vi "FPGA car.vi"() -> ()   [LabVIEW 2019]
doc: "The myRIO v1.1 FPGA Shipping Personality. This personality contains support for:\n- 2 Analog Input Interrupt channel\n- 4 Digital Input Interrupt channel\n- 1 Timer\n- 1 Accelerometer\n- 1 Button\n- 4 LED\n- 10 Analog Input channels with 1 Sample\n- 6 Analog Output channels with 1 Sample\n- 40 Digital I/O channels with 1 Sample\n- 2 I2C channels\n- 4 Encoder channels\n- 6 PWM channels\n- 2 SPI channels"
uses:
  Sub VIs/Utilities/Start Boolean.ctl
  <vilib>/Platform/TimedLoop/XDataNode/timing_clust.ctl
  <vilib>/Platform/TimedLoop/XDataNode/nitl_modes.ctl
  <vilib>/Platform/TimedLoop/XDataNode/wakeup.ctl
  <vilib>/rvi/Emulation/niFpgaGetClockAttributes.vi
  <vilib>/rvi/Emulation/niFpgaSctlEmulationGetInTimedLoop.vi
  <vilib>/rvi/Emulation/niFpgaEmulationReportErrorSimple.vi
  <vilib>/rvi/eio/common/nirviEmuTemplateMethod_errors.vi
  <vilib>/rvi/Emulation/niFpgaProcessEmulError.vi
  <vilib>/rvi/Emulation/niFpgaCriticalErrorInLSC.vi
  <vilib>/eio/EIONode/EIONode.xnode
  <vilib>/Platform/TimedLoop/XDataNode/XDataNode.xnode
  <vilib>/Platform/TimedLoop/XDataNode/XDNodeRunTimeDep.lvlib
panel:
  out "Position 4":i32
  in  "Direction 2":bool
  in  "puls duration us (0-2^16) 2":u32
  in  "Reset 4":bool
  out "Position 3":i32
  in  "Direction":bool
  in  "puls duration us (0-2^16)":u32
  in  "Reset 3":bool
  out "Position 2":i32
  out "Position":i32
  out "arrived 2":bool
  in  "Max_speed half period (us) 2":u16
  in  "Acceleration 2":u16
  in  "Min_speed half period (us) 2":u16
  in  "Soll_pos (Halbschritte) 2":i32
  in  "Reset 2":bool
  out "arrived":bool
  in  "Acceleration":u16
  in  "Max_speed half period (us)":u16
  in  "Min_speed half period (us)":u16
  in  "Reset":bool
  in  "Soll_pos (Halbschritte)":i32
  in  "Duty_counts (0-40)":u16 caption="Count(uSec)"
  out "Time1":u16
  out "Time2":u16
  out "Time 3":u16
  in  "Timeout US":u16
  in  "DO.LED3:0":u8 format="%04b"
  in  "DIO.A_15:8.DIR":u8 format="%08b"
  in  "DIO.A_15:8.OUT":u8 format="%08b"
  in  "SYS.SELECTA":u8 format="%08b"
  out "DIO.A_15:8.IN":u8 format="%08b"
  in  "PWM 2 value (0-1000)":u16
  in  "PWM 1 value (0-1000)":u16
  in  "PWM 0 value (0-1000)":u16
  out "PulseWidth 3":u16
  out "PulseWidth 2":u16
  out "PulseWidth 1":u16
  out "I2C.A.STAT":u8 format="%08b"
  in  "I2C.A.CNTL":u8 format="%08b"
  in  "I2C.A.CNTR":u8=213
  in  "I2C.A.ADDR":u8 format="%08b"
  out "I2C.A.DATI":u8
  in  "I2C.A.DATO":u8
  in  "I2C.A.CNFG":u8=1 format="%08b"
  in  "I2C.A.GO":T1
  out "SYS.AI.RDY":bool
  out "SYS.RDY":bool
  out "ACC.X.VAL":u16
  out "ACC.Y.VAL":u16
  out "SYS.ACC.RDY":bool
  out "ACC.Z.VAL":u16
  # "System"
  # "Onboard Devices"
  # "Connector A"
  # "Accelerometer"
  # "Analog Input"
  # "PWM Output"
  # "PW_Measurement"
  # "I2C Master"
  # "US Measurements"
  # "Stepper Speed"
  # "Stepper Position Freq/Dir"
  # "Led"
  # "Lidar"
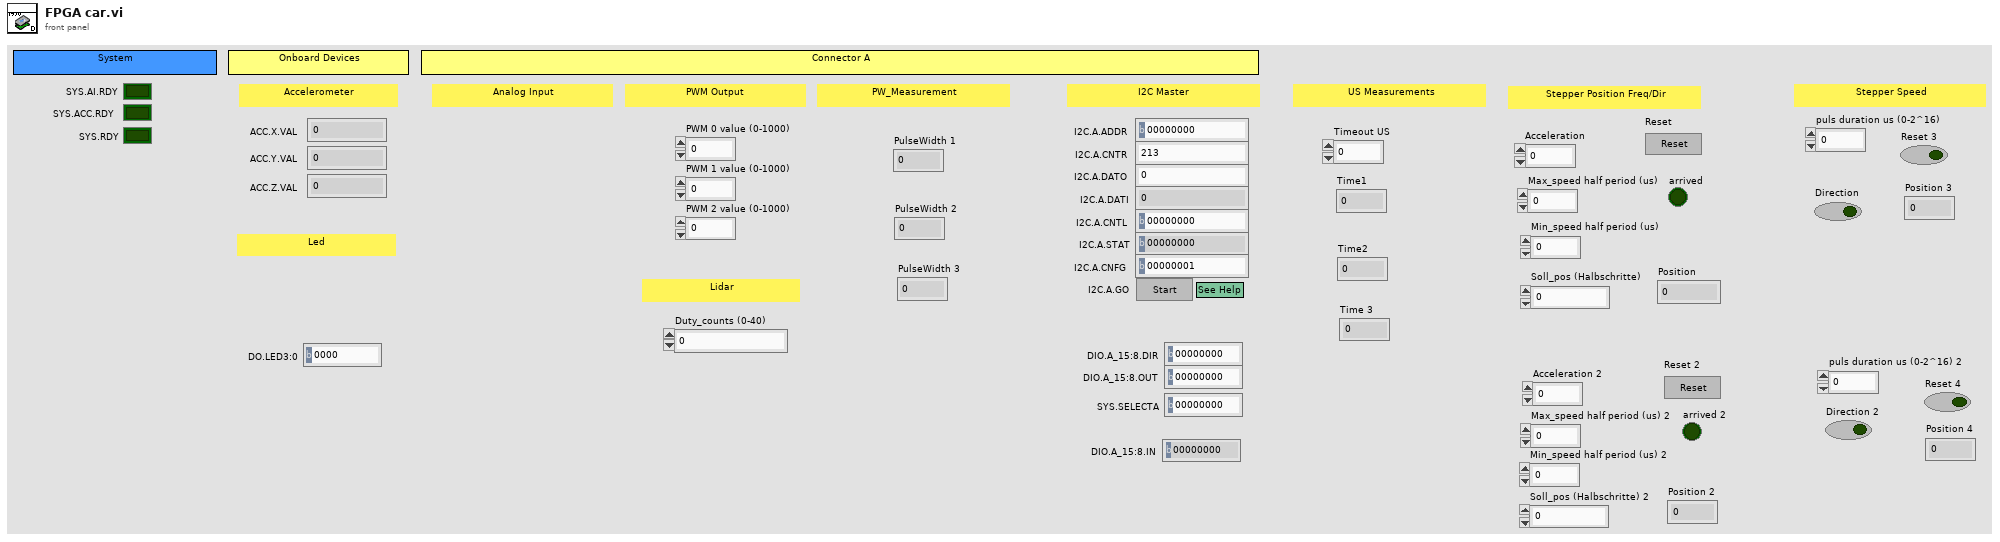
[diagram p1: front panel]
types:
  T1 = typedef "Start Boolean.ctl" = bool
  T2 = typedef "XDNodeRunTimeDep.lvlib/timing_clust.ctl" = cluster{"Expected End [f-1]":u64, "Actual End [f-1]":u64, "Finished Late? [f-1]":bool, "Expected End [i-1]":u64, "Actual End [i-1]":u64, "Finished Late? [i-1]":bool, "Expected Start [i]":u64, "Actual Start [i]":u64, "Expected Start [f]":u64, "Actual Start [f]":u64, "Source Name":string, "Structure Name":string, "Period":i64, "Deadline":i64, "Offset":i64, "Start":i64, "Priority":i32, "Timeout":i32, "Mode":T3, "Wakeup Reason":T4, "Error":errorcluster, "Source Type":string, "Secondary Source Type":string, "Global End Time":u64, "Global Start Time":u64, "Frame Duration":u64, "Iteration Duration":u64, "Assigned CPU":i32, "I/O Scan Engine Mode":u32}
  T3 = typedef "XDNodeRunTimeDep.lvlib/nitl_modes.ctl" = enum32{"No Change", "Process missed periods, maintain original phase", "Discard missed periods, maintain original phase", "Process missed periods, ignore original phase", "Discard missed periods, ignore original phase"}
  T4 = typedef "XDNodeRunTimeDep.lvlib/wakeup.ctl" = enum32{"Normal", "Aborted", "Asynchronous wakeup", "Timing source error", "Timed loop error", "Timeout"}
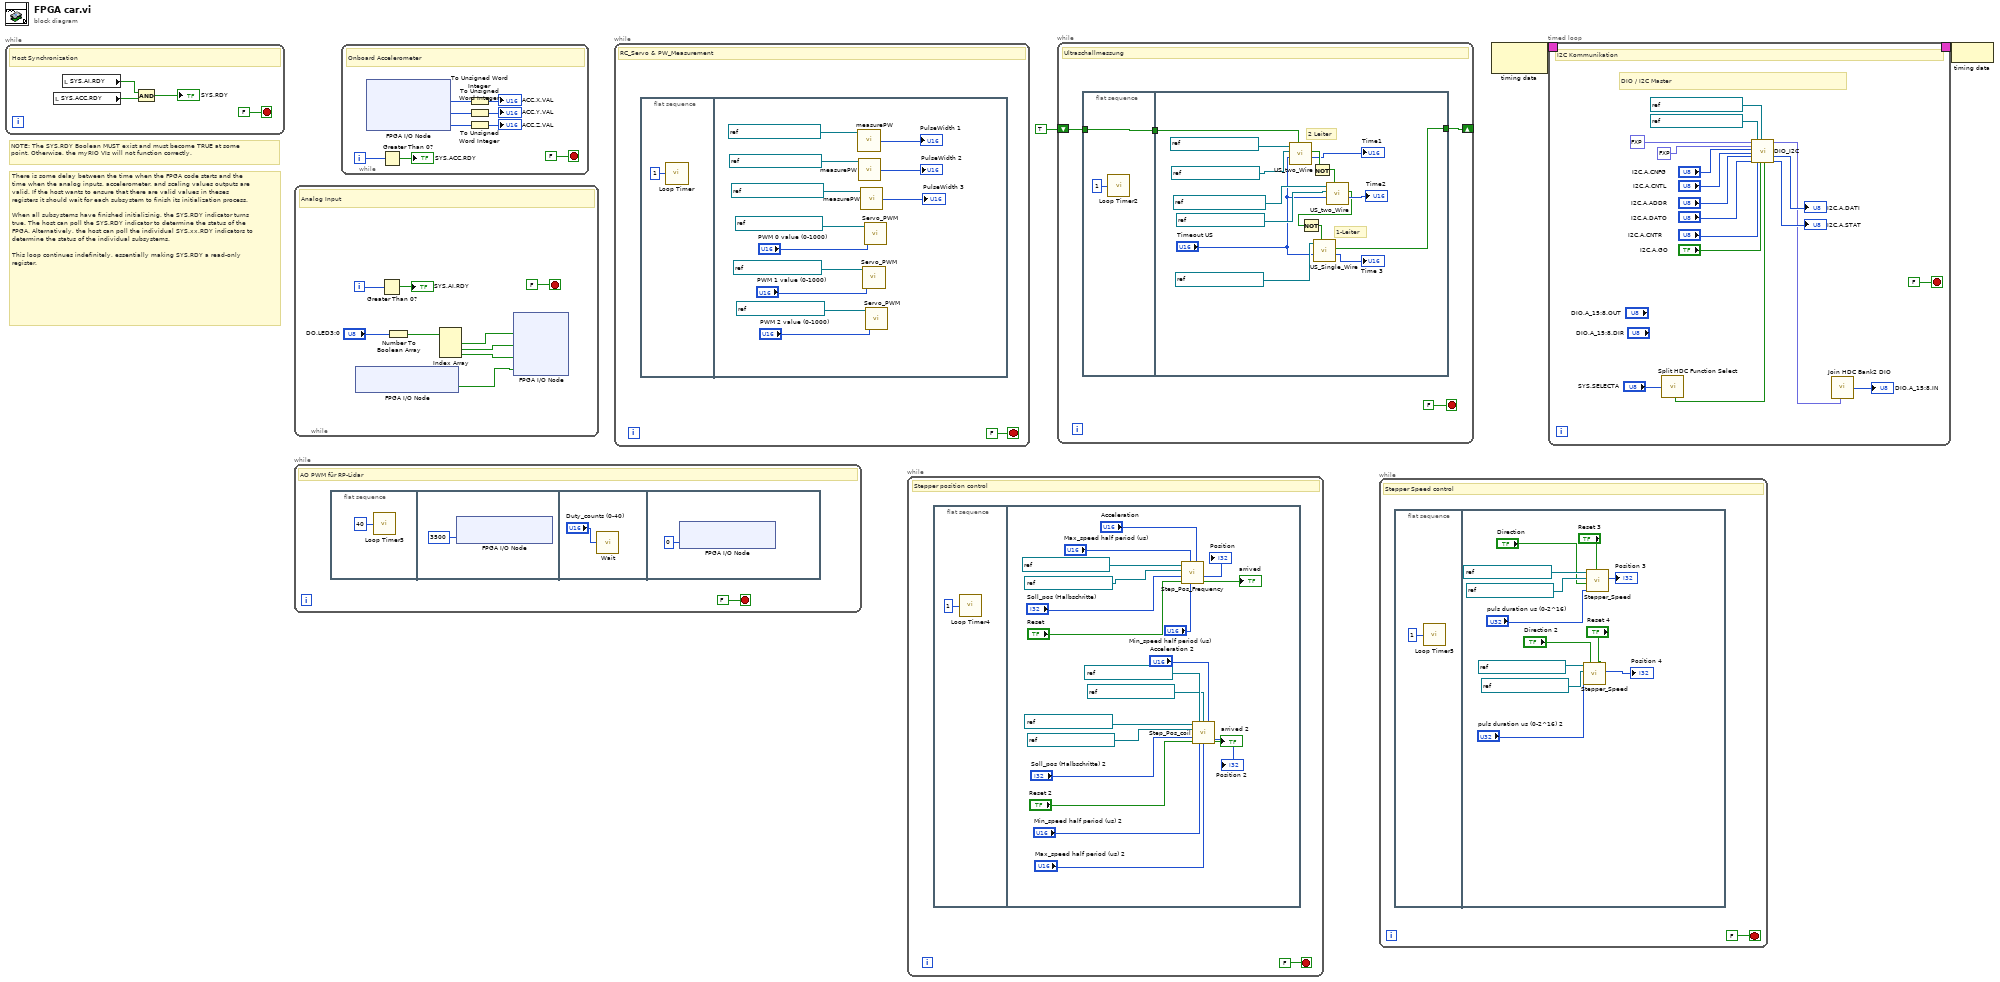
[diagram p0: block diagram]
diagram:
  # "NOTE: The SYS.RDY Boolean MUST exist and must become TRUE at some point. Otherwise, the myRIO VIs will not function correctly."
  # "There is some delay between the time when the FPGA code starts and the time when the analog inputs, accelerometer, and scaling values outputs are valid. If the host wants to ensure that there are valid values in theses registers it should wait for each subsystem to finish its initialization process. \n\nWhen all subsystems have finished initializinig, the SYS.RDY indicator turns true. The host can poll the SYS.RDY indicator to determine the status of the FPGA. Alternatively, the host can poll the individual SYS.xx.RDY indicators to determine the status of the individual subsystems.\n\nThis loop continues indefinitely, essentially making SYS.RDY a read-only register."
  n1 = while {
    stop <- FALSE stop-if-true
    # "Host Synchronization"
    n2 = local read "SYS.ACC.RDY"() -> (w5:bool)
    n3 = local read "SYS.AI.RDY"() -> (w7:bool)
    n4 = Compound Arithmetic op=AND(w7, w5) -> (→"SYS.RDY":bool)
  }
  n5 = while {
    stop <- FALSE stop-if-true
    # "AO PWM für RP-Lidar"
    n6 = flat-sequence {
      frame #0 {
        n7 = call "Loop Timer3"("Count(uSec)"=u16 40) -> ()  [unwired: 1 out]
      }
      frame #1 {
        n8 = xnode "FPGA I/O Node"("ConnectorB/AO0"=u16 3500) -> ()  [unwired: 1 in, 1 out]
      }
      frame #2 {
        n9 = call "Wait"("Count(uSec)"="Duty_counts (0-40)") -> ()  [unwired: 1 out]
      }
      frame #3 {
        n10 = xnode "FPGA I/O Node"("ConnectorB/AO0"=u16 0) -> ()  [unwired: 1 in, 1 out]
      }
    }
  }
  n11 = while {
    i -> [w20]
    stop <- FALSE stop-if-true
    # "Analog Input"
    n12 = xnode "FPGA I/O Node"() -> ("ConnectorA/DIO10"=w13:bool)  [unwired: 1 in, 1 out]
    n13 = Greater Than 0?(x=w20) -> (x > 0?=→"SYS.AI.RDY":bool)
    n14 = Number To Boolean Array(number="DO.LED3:0") -> (Boolean array=w17:bool[])
    n15 = Index Array(array=w17) -> (element #1=w16:bool, element #2=w15:bool, element #3=w14:bool)  [unwired: 3 in]
    n16 = xnode "FPGA I/O Node"("LED0"=w16, "LED1"=w15, "LED2"=w14, "LED3"=w13) -> ()  [unwired: 4 in, 4 out]
  }
  n17 = while {
    i -> [w26]
    stop <- FALSE stop-if-true
    # "Onboard Accelerometer"
    n18 = xnode "FPGA I/O Node"() -> ("AccelerationX"=w29:i16, "AccelerationY"=w28:i16, "AccelerationZ"=w27:i16)  [unwired: 3 in, 3 out]
    n19 = Greater Than 0?(x=w26) -> (x > 0?=→"SYS.ACC.RDY":bool)
    n20 = To Unsigned Word Integer(number=w29) -> (unsigned 16bit integer=→"ACC.X.VAL":u16)
    n21 = To Unsigned Word Integer(number=w28) -> (unsigned 16bit integer=→"ACC.Y.VAL":u16)
    n22 = To Unsigned Word Integer(number=w27) -> (unsigned 16bit integer=→"ACC.Z.VAL":u16)
  }
  n23 = while {
    stop <- FALSE stop-if-true
    # "RC_Servo & PW_Measurement"
    n24 = flat-sequence {
      frame #0 {
        n25 = call "Loop Timer"("Count(uSec)"=u16 1 ("Count(Ticks)")) -> ()  [unwired: 1 out]
      }
      frame #1 {
        n26 = call "measurePW.vi"("Refnum in"=refnum<k21> "ConnectorA/DIO11" ("DIO/PWM")) -> ("value"=→"PulseWidth 1":u16)  [unwired: 10 in]
        n27 = call "measurePW.vi"("Refnum in"=refnum<k21> "ConnectorA/DIO12" ("DIO/PWM")) -> ("value"=→"PulseWidth 2":u16)  [unwired: 10 in]
        n28 = call "measurePW.vi"("Refnum in"=refnum<k21> "ConnectorA/DIO13" ("DIO/PWM")) -> ("value"=→"PulseWidth 3":u16)  [unwired: 10 in]
        n29 = call "Servo_PWM.vi"("value (0-1000)"="PWM 1 value (0-1000)", "Refnum in"=refnum<k21> "ConnectorA/DIO1" ("DIO/PWM")) -> ()  [unwired: 10 in]
        n30 = call "Servo_PWM.vi"("value (0-1000)"="PWM 0 value (0-1000)", "Refnum in"=refnum<k21> "ConnectorA/DIO0" ("DIO/PWM")) -> ()  [unwired: 10 in]
        n31 = call "Servo_PWM.vi"("value (0-1000)"="PWM 2 value (0-1000)", "Refnum in"=refnum<k21> "ConnectorA/DIO2" ("DIO/PWM")) -> ()  [unwired: 10 in]
      }
    }
  }
  n32 = while {
    stop <- FALSE stop-if-true
    # "Stepper position control"
    n33 = flat-sequence {
      frame #0 {
        n34 = call "Loop Timer4"("Count(uSec)"=u16 1 ("Count(Ticks)")) -> ()  [unwired: 1 out]
      }
      frame #1 {
        n35 = call "Step_Pos_Frequency.vi"("Acceleration"="Acceleration", "Min_speed half period (us)"="Min_speed half period (us)", "Max_speed half period (us)"="Max_speed half period (us)", "Reset"="Reset", "Soll_pos (Halbschritte)"="Soll_pos (Halbschritte)", "DO_Direction"=refnum<k21> "ConnectorB/DIO1" ("DIO/PWM"), "DO_Frequency"=refnum<k21> "ConnectorB/DIO0" ("DIO/PWM")) -> ("arrived"=→"arrived":bool, "Position"=→"Position":i32)  [unwired: 1 in, 2 out]
        n36 = call "Step_Pos_coil.vi"("DO_C1_1"=refnum<k21> "ConnectorB/DIO2" ("DIO/PWM"), "DO_C2_1"=refnum<k21> "ConnectorB/DIO4" ("DIO/PWM"), "DO_C2_2"=refnum<k21> "ConnectorB/DIO5" ("DIO/PWM"), "Acceleration"="Acceleration 2", "DO_C1_2"=refnum<k21> "ConnectorB/DIO3" ("DIO/PWM"), "Soll_pos (Halbschritte)"="Soll_pos (Halbschritte) 2", "Reset"="Reset 2", "Min_speed half period (us)"="Min_speed half period (us) 2", "Max_speed half period (us)"="Max_speed half period (us) 2") -> ("Position"=→"Position 2":i32, "arrived"=→"arrived 2":bool)  [unwired: 1 in, 4 out]
      }
    }
  }
  n37 = while {
    shift-right: [w67] -> _
    shift-left: TRUE -> [w69]
    stop <- FALSE stop-if-true
    # "Ultraschallmessung"
    n38 = flat-sequence {
      tunnel: w69 -> [w71]
      tunnel: [w71] -> w68
      tunnel: w68 -> [w85]
      tunnel: [w73] -> w67
      frame #0 {
        n39 = call "Loop Timer2"("Count(uSec)"=u16 1 ("Count(Ticks)")) -> ()  [unwired: 1 out]
      }
      frame #1 {
        # "1-Leiter"
        # "2 Leiter"
        n40 = call "US_two_Wire.vi"("start ping"=w85, "Timeout (usec)"="Timeout US", "Echo_Line"=refnum<k21> "ConnectorA/DIO6" ("DIO/PWM"), "Ping_Line"=refnum<k21> "ConnectorA/DIO5" ("DIO/PWM")) -> ("echo_time(us)"=→"Time1":u16, "busy"=w83:bool)  [unwired: 6 in]
        n41 = Not(x=w83) -> (.not. x?=w84:bool)
        n42 = call "US_two_Wire.vi"("start ping"=w84, "Timeout (usec)"="Timeout US", "Echo_Line"=refnum<k21> "ConnectorA/DIO0" ("DIO/PWM"), "Ping_Line"=refnum<k21> "ConnectorA/DIO13" ("DIO/PWM")) -> ("echo_time(us)"=→"Time2":u16, "busy"=w78:bool)  [unwired: 6 in]
        n43 = Not(x=w78) -> (.not. x?=w77:bool)
        n44 = call "US_Single_Wire.vi"("start ping"=w77, "Timeout (usec)"="Timeout US", "Refnum in"=refnum<k21> "ConnectorA/DIO1" ("DIO/PWM")) -> ("echo_time(us)"=→"Time 3":u16, "busy"=w73:bool)  [unwired: 7 in]
      }
    }
  }
  n45 = while {
    stop <- FALSE stop-if-true
    # "Stepper Speed control"
    n46 = flat-sequence {
      frame #0 {
        n47 = call "Loop Timer5"("Count(uSec)"=u16 1 ("Count(Ticks)")) -> ()  [unwired: 1 out]
      }
      frame #1 {
        n48 = call "Stepper_Speed.vi"("Reset"="Reset 4", "puls duration us (0-2^16)"="puls duration us (0-2^16) 2", "Direction"="Direction 2", "Direction Pin"=refnum<k21> "ConnectorB/DIO5" ("DIO/PWM"), "PWM Pin"=refnum<k21> "ConnectorB/DIO4" ("DIO/PWM")) -> ("Position"=→"Position 4":i32)  [unwired: 2 in]
        n49 = call "Stepper_Speed.vi"("Reset"="Reset 3", "puls duration us (0-2^16)"="puls duration us (0-2^16)", "Direction"="Direction", "Direction Pin"=refnum<k21> "ConnectorB/DIO5" ("DIO/PWM"), "PWM Pin"=refnum<k21> "ConnectorB/DIO4" ("DIO/PWM")) -> ("Position"=→"Position 3":i32)  [unwired: 2 in]
      }
    }
  }
  n50 = node-c288() -> (w3:T2)  [unwired: 1 in]
  n51 = timed-loop {
    timing: w3 -> [_]
    timing-out: [_] -> w2
    stop <- FALSE stop-if-true
    # "DIO / I2C Master"
    # "I2C Kommunikation"
    n52 = call "Split HDC Function Select.vi"("IN 7:0"="SYS.SELECTA") -> ("OUT 7"=w102:bool)  [unwired: 5 out]
    n53 = call "DIO_I2C.vi"("DIO.1:0.OUT"=fxp<+,2,2> 0.0 ("OUT 7:6"), "DIO.1:0.DIR"=fxp<+,2,2> 0.0 ("OUT 7:6"), "I2C.CNFG"="I2C.A.CNFG", "I2C.CNTL"="I2C.A.CNTL", "I2C.ADDR"="I2C.A.ADDR", "I2C.DATO"="I2C.A.DATO", "DIO.1/I2C.SDA"=refnum<k21> "ConnectorA/DIO15" ("DIO.1/I2C.SCL"), "I2C.CNTR"="I2C.A.CNTR", "DIO.0/I2C.SCL"=refnum<k21> "ConnectorA/DIO14" ("DIO.0/I2C.SDA"), "Execute?"="I2C.A.GO", "SELECT"=w102) -> ("DIO.1:0.IN"=w104:fxp<+,2,2>, "I2C.DATI"=→"I2C.A.DATI":u8, "I2C.STAT"=→"I2C.A.STAT":u8)  [unwired: 6 in]
    n54 = call "Join HDC Bank2 DIO.vi"("IN 7:6"=w104) -> ("OUT 7:0"=→"DIO.A_15:8.IN":u8)  [unwired: 9 in]
  }
  n55 = node-c288(w2) -> ()
